vi "to_deg_F_subVI.vi"(11 "Bytes Read":u8[](array[numeric])) -> (3 "Numeric":dbl)   [LabVIEW 2021]
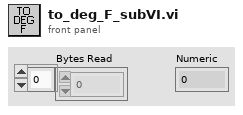
[diagram p1: front panel]
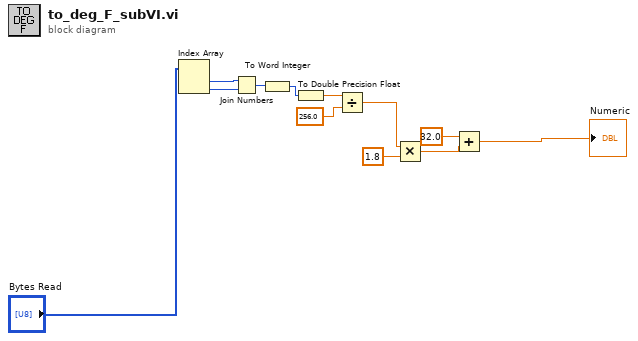
[diagram p0: block diagram]
diagram:
  n1 = Index Array(array="Bytes Read") -> (element #1=w6:u8, element #2=w7:u8)  [unwired: 2 in]
  n2 = Join Numbers(hi=w6, lo=w7) -> ((hi.lo)=w4:u16)
  n3 = To Word Integer(number=w4) -> (16bit integer=w1:i16)
  n4 = To Double Precision Float(number=w1) -> (double precision float=w2:dbl)
  n5 = Divide(x=w2, y=256.0) -> (x/y=w8:dbl)
  n6 = Multiply(x=w8, y=1.8) -> (x*y=w10:dbl)
  n7 = Add(x=32.0, y=w10) -> (x+y=→"Numeric":dbl)
